vi "Get Channel Value.vi"(8 "error in":errorcluster, 10 "Data Reference in":T1 format="%.0x", 11 "VS Engine in":refnum<class "VS Engine.lvclass">=refnum) -> (0 "error out":errorcluster, 2 "Value":dbl, 3 "VS Engine out":refnum<class "VS Engine.lvclass">)   [LabVIEW 2024, in "VS Engine Abstraction.lvlib" / "VS Engine.lvclass"]
uses:
  VS Engine.lvclass
  VS Engine.lvclass/VS Engine.ctl
  <vilib>/NI VeriStand/Custom Device API/Custom Device API.lvlib
  <vilib>/NI VeriStand/Custom Device API/Data Reference.ctl
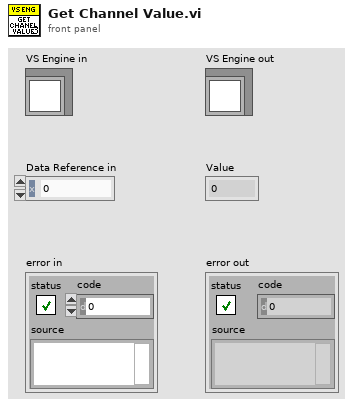
[diagram p1: front panel]
types:
  T1 = typedef "Custom Device API.lvlib/Data Reference.ctl" = i32
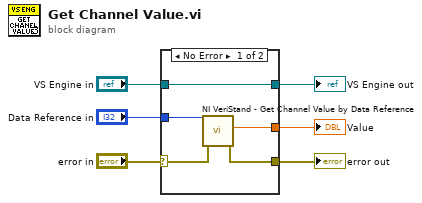
[diagram p0: block diagram]
diagram:
  n1 = case shown="No Error" "error in" {
    selector: "error in" -> [w11 w13]
    tunnel: [w9 _] -> w4
    tunnel: "Data Reference in" -> [w8 _]
    tunnel: [w10 w13] -> w5
    tunnel: [w7 w12] -> w1
    tunnel: "VS Engine in" -> [w7 w12]
    frame No Error {
      n2 = call <vilib>:"NI VeriStand - Get Channel Value by Data Reference.vi"("error in (no error)"=w11, "Data Reference in"=w8) -> ("error out"=w10:errorcluster, "Value"=w9:dbl)  [unwired: 8 in]
    }
    frame Error {
    }
  }
  "error out" <- w5
  "VS Engine out" <- w1
  "Value" <- w4
